vi "Update Icon if New Class.vi"(8 "error in (no error)":errorcluster, 9 "Label BG Color":u32(colorbox)=16765344, 10 "New Name":string="Test", 11 "Library Refnum In":refnum<vi>) -> (0 "error out":errorcluster, 3 "Library Refnum Out":refnum<vi>)   [LabVIEW 2020, in "ADAS_IO_Template_MDO.lvclass"]
uses:
  ADAS_IO_Template_MDO.lvclass
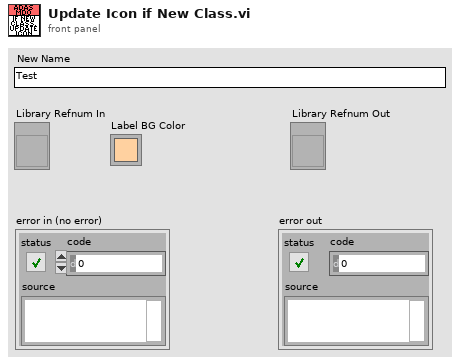
[diagram p1: front panel]
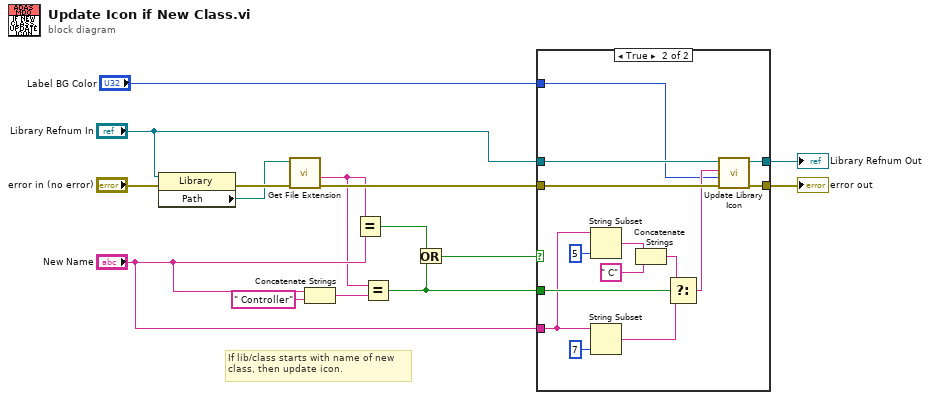
[diagram p0: block diagram]
diagram:
  # "If lib/class starts with name of new\nclass, then update icon."
  n1 = property class="Library"(reference="Library Refnum In", error in="error in (no error)") -> (error out=w12:errorcluster, "Path"=w10:path)  [unwired: 1 out]
  n2 = call <vilib>:"Get File Extension.vi"("error in (no error)"=w12, "file"=w10) -> ("error out"=w11:errorcluster, "filename without extension"=w6:string)  [unwired: 5 in, 3 out]
  n3 = Concatenate Strings("New Name", " Controller" ("string")) -> (w7:string)
  n4 = Equal?(x=w6, y="New Name") -> (x = y?=w2:bool)
  n5 = Equal?(x=w6, y=w7) -> (x = y?=w3:bool)
  n6 = Or(x=w2, y=w3) -> (x .or. y?=w5:bool)
  n7 = case shown="True" w5 {
    tunnel: w11 -> [w17 w31]
    tunnel: "New Name" -> [_ w22]
    tunnel: [w16 w29] -> w14
    tunnel: [w17 w28] -> w13
    tunnel: "Library Refnum In" -> [w16 w27]
    tunnel: w3 -> [_ w26]
    tunnel: "Label BG Color" -> [_ w18]
    frame False {
    }
    frame True {
      n8 = String Subset(string=w22, length (rest)=5 ("length (rest)")) -> (substring=w21:string)  [unwired: 1 in]
      n9 = String Subset(string=w22, length (rest)=7 ("length (rest)")) -> (substring=w25:string)  [unwired: 1 in]
      n10 = Concatenate Strings(w21, " C" ("t")) -> (w19:string)
      n11 = Select(t=w19, s=w26, f=w25) -> (s? t:f=w24:string)
      n12 = call "Update Library Icon.vi"("error in (no error)"=w31, "Label BG Color"=w18, "Label Text"=w24, "Library Refnum in"=w27) -> ("error out"=w28:errorcluster, "Library Refnum Out"=w29:refnum<vi>)  [unwired: 6 in]
    }
  }
  "Library Refnum Out" <- w14
  "error out" <- w13
